vi "Camera_Config.vi"(5 "Crop?":bool, 6 "Camera":T5, 7 "error in":errorcluster, 8 "input cluster":T1={"L16 Linear Actuator"="", "XE 1000 Pump"="", "Camera1"="", "Camera2"="", "Img_Capt"=FALSE, "Actuator"=FALSE, "Pump"=FALSE, "Cam 1"=FALSE, "Cam 2"=FALSE, "Empty_Refill"=FALSE, "Crop"=FALSE, "Light intensity"=100, "Exposure Time"=1000.0, "Sample Name"="Test Sample", "Operator"="MRJ", "Calibration 1"=path "C:/Users/au540322/Desktop/IHS_Project/images/Debris/Debris_0/Debris_0_2019_06_01-23-32-49-686.PNG", "Calibration 2"=path "C:/Users/au540322/Desktop/IHS_Project/images/Debris/Debris_0/Debris_0_2019_06_01-23-32-49-686.PNG", "Framerate"=1, "Timeout Sample"=0, "Collection date"="MRJ", "Sample size threshold"=1, "Empty start"=1, "Command"="MRJ", "Station"="", "Species Name"="", "Other Notes"="", "Aperture"=enum."Item 0", "Image Process Queue Size"=500, "Image Save Queue Size"=500, "Overload threshold"=500, "Max Framerate"=100, "Rectangle 1"={"Left"=0, "Top"=0, "Right"=0, "Bottom"=0, "Rotation"=0.0}, "Rectangle 2"={"Left"=0, "Top"=0, "Right"=0, "Bottom"=0, "Rotation"=0.0}, "Detection Region %"=0.0, "Detect 1"=path "C:/Users/au540322/Desktop/IHS_Project/images/Debris/Debris_0/Debris_0_2019_06_01-23-32-49-686.PNG", "Detect 2"=path "C:/Users/au540322/Desktop/IHS_Project/images/Debris/Debris_0/Debris_0_2019_06_01-23-32-49-686.PNG", "Max large object threshold"=0, "Open(T)/Close(F)"=FALSE, "Img_Capt Begin"=FALSE, "Dispense Speed"=100, "Flush Size"=100, "Location"="Station", "Latitude"="Station", "Longitude"="Station", "Determiner"="Station", "Sex"="Station", "Camera1_Img"=refnum, "Camera2_Img"=refnum, "Img1_Orig_Disp"=refnum, "Img2_Orig_Disp"=refnum, "Img1_Orig_RGB"=refnum, "Img2_Orig_RGB"=refnum, "Blue_Plane_Extract"=refnum, "Subtracted_Plane"=refnum, "Img1_Binary"=refnum, "Img2_Binary"=refnum, "Crop_Mask"=refnum, "Img1_Save"=refnum, "Img2_Save"=refnum, "Img1_Cali_Full"=refnum, "Img2_Cali_Full"=refnum, "Img1_Cali_Detect"=refnum, "Img2_Cali_Detect"=refnum, "Cam 1 queue"=refnum, "Cam 2 queue"=refnum, "Cam 1 - save queue"=refnum, "Cam 2 - save queue"=refnum, "Overlay_Ring"=0, "SystemVersion"=0, "System Serial"=""} {"SystemVersion" items=["Standard", "XL"]; "Overlay_Ring" items=["Session Data", "Extended Setup", "Buffer", "Camera", "Dispenser", "Stats", "Connections"]; "Flush Size" min=1; "Dispense Speed" min=1; "Rectangle 2"."Rotation" format="%.2f"; "Rectangle 2"."Left" scale=0.0..1024.0; "Rectangle 2"."Right" scale=0.0..1024.0; "Rectangle 1"."Rotation" format="%.2f"; "Rectangle 1"."Left" scale=0.0..1024.0; "Rectangle 1"."Right" scale=0.0..1024.0; "Max Framerate" min=1; "Overload threshold" min=1; "Image Save Queue Size" min=1; "Image Process Queue Size" min=1; "Empty start" min=1; "Sample size threshold" min=1; "Framerate" min=1; "Light intensity" scale=0.0..100.0}, 9 "Detect Movement":bool, 10 "Refnum in":T2="cam2") -> (0 "error out":errorcluster, 3 "Refnum out":T2="cam2")   [LabVIEW 2021]
doc: "Configures basler cameras for image acquisition with cropped aspectratio."
uses:
  <vilib>/userDefined/High Color/IMAQdx.ctl
  Camera_ID.ctl
  controls/Data.ctl
  <vilib>/vision/Image Controls.llb/IMAQ Image.ctl
  <resource>/objmgr/imaqdx.rc
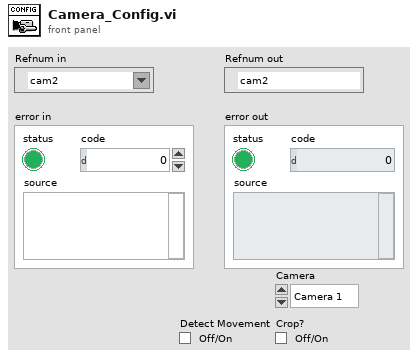
[diagram p1: front panel]
types:
  T1 = typedef "Data.ctl" = cluster{"L16 Linear Actuator":refnum<visa-resource-name>, "XE 1000 Pump":refnum<visa-resource-name>, "Camera1":T2, "Camera2":T2, "Img_Capt":bool, "Actuator":bool, "Pump":bool, "Cam 1":bool, "Cam 2":bool, "Empty_Refill":bool, "Crop":bool, "Light intensity":i32, "Exposure Time":dbl, "Sample Name":string, "Operator":string, "Calibration 1":path, "Calibration 2":path, "Framerate":i32, "Timeout Sample":i32, "Collection date":string, "Sample size threshold":i32, "Empty start":u32, "Command":string, "Station":string, "Species Name":string, "Other Notes":string, "Aperture":enum32{"Item 0", "Item 1", "Item 2", "Item 3"}, "Image Process Queue Size":i32, "Image Save Queue Size":i32, "Overload threshold":i32, "Max Framerate":i32, "Rectangle 1":T3, "Rectangle 2":T3, "Detection Region %":dbl, "Detect 1":path, "Detect 2":path, "Max large object threshold":i32, "Open(T)/Close(F)":bool, "Img_Capt Begin":bool, "Dispense Speed":i32, "Flush Size":i32, "Location":string, "Latitude":string, "Longitude":string, "Determiner":string, "Sex":string, "Camera1_Img":T4, "Camera2_Img":T4, "Img1_Orig_Disp":T4, "Img2_Orig_Disp":T4, "Img1_Orig_RGB":T4, "Img2_Orig_RGB":T4, "Blue_Plane_Extract":T4, "Subtracted_Plane":T4, "Img1_Binary":T4, "Img2_Binary":T4, "Crop_Mask":T4, "Img1_Save":T4, "Img2_Save":T4, "Img1_Cali_Full":T4, "Img2_Cali_Full":T4, "Img1_Cali_Detect":T4, "Img2_Cali_Detect":T4, "Cam 1 queue":refnum<queue>, "Cam 2 queue":refnum<queue>, "Cam 1 - save queue":refnum<queue>, "Cam 2 - save queue":refnum<queue>, "Overlay_Ring":u16, "SystemVersion":u16, "System Serial":string}
  T2 = typedef "IMAQdx.ctl" = refnum<k21>
  T3 = typedef "IMAQ Rectangle" = cluster{"Left":i32, "Top":i32, "Right":i32, "Bottom":i32, "Rotation":dbl}
  T4 = typedef "IMAQ Image.ctl" = refnum<image>
  T5 = typedef "Camera_ID.ctl" = enum16{"Camera 1", "Camera 2"}
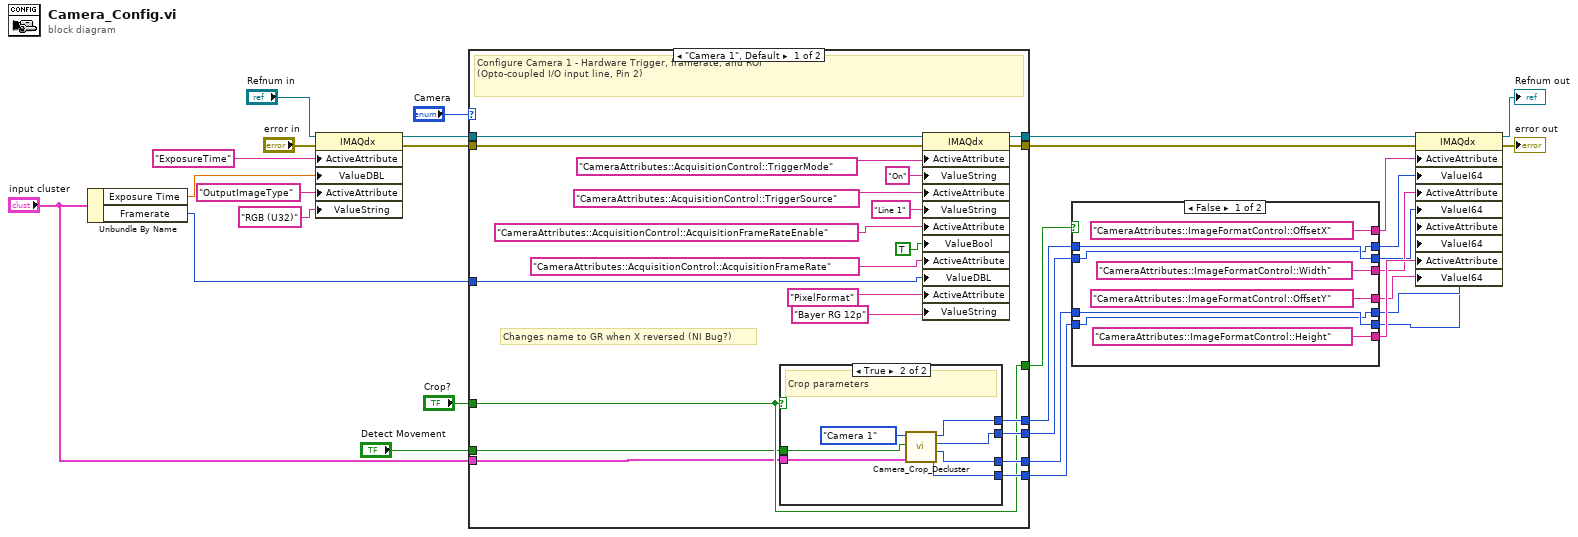
[diagram p0: block diagram]
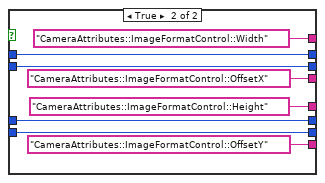
[diagram p2: hidden frame]
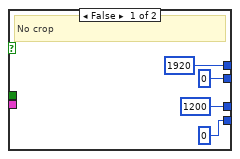
[diagram p3: hidden frame]
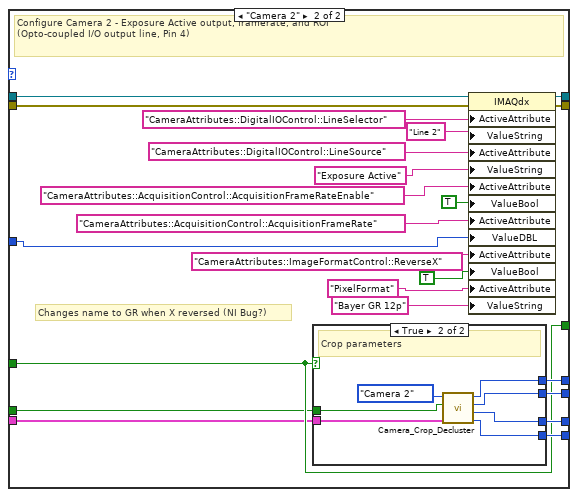
[diagram p4: hidden frame]
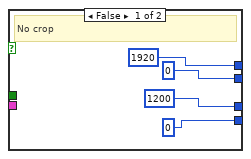
[diagram p5: hidden frame]
diagram:
  n1 = Unbundle By Name("input cluster") -> ("Exposure Time"=w28:dbl, "Framerate"=w27:i32)
  n2 = property class="IMAQdx"(reference="Refnum in", error in="error in", "ActiveAttribute"="ExposureTime", "ValueDBL"=w28, "ActiveAttribute"="OutputImageType", "ValueString"="RGB (U32)") -> (reference out=w21:T2, error out=w3:errorcluster)
  n3 = case shown="\"Camera 1\", Default" "Camera" {
    tunnel: w21 -> [w51 w72]
    tunnel: [w50 w71] -> w19
    tunnel: [w49 w70] -> w26
    tunnel: w27 -> [w41 w69]
    tunnel: [w39 w85] -> w13
    tunnel: [w40 w84] -> w16
    tunnel: [w37 w82] -> w11
    tunnel: [w38 w83] -> w15
    tunnel: "Crop?" -> [w36 w81]
    tunnel: [w36 w81] -> w18
    tunnel: "input cluster" -> [w35 w80]
    tunnel: "Detect Movement" -> [w34 w79]
    tunnel: w3 -> [w33 w65]
    frame "Camera 1", Default {
      # "Changes name to GR when X reversed (NI Bug?)"
      # "Configure Camera 1 - Hardware Trigger, framerate, and ROI \n(Opto-coupled I/O input line, Pin 2)"
      n4 = case shown="True" w36 {
        tunnel: [i64 1920 w61] -> w40
        tunnel: [1200 w59] -> w39
        tunnel: [i64 0 w60] -> w38
        tunnel: [0 w58] -> w37
        tunnel: w35 -> [_ w57]
        tunnel: w34 -> [_ w56]
        frame False {
          # "No crop"
        }
        frame True {
          # "Crop parameters"
          n5 = call "Camera_Crop_Decluster.vi"("input cluster"=w57, "Detect Movement"=w56, "Camera"=Camera_ID."Camera 1") -> ("OffsetY"=w58:i64, "Height"=w59:i64, "OffsetX"=w60:i64, "Width"=w61:i64)  [unwired: 5 in]
        }
      }
      n6 = property class="IMAQdx"(reference=w51, error in=w33, "ActiveAttribute"="CameraAttributes::AcquisitionControl::TriggerMode", "ValueString"="On", "ActiveAttribute"="CameraAttributes::AcquisitionControl::TriggerSource", "ValueString"="Line 1", "ActiveAttribute"="CameraAttributes::AcquisitionControl::AcquisitionFrameRateEnable", "ValueBool"=TRUE, "ActiveAttribute"="CameraAttributes::AcquisitionControl::AcquisitionFrameRate", "ValueDBL"=w41, "ActiveAttribute"="PixelFormat", "ValueString"="Bayer RG 12p") -> (reference out=w50:T2, error out=w49:errorcluster)
    }
    frame "Camera 2" {
      # "Changes name to GR when X reversed (NI Bug?)"
      # "Configure Camera 2 - Exposure Active output, framerate, and ROI\n(Opto-coupled I/O output line, Pin 4)"
      n7 = case shown="True" w81 {
        tunnel: [i64 1200 w92] -> w85
        tunnel: [i64 1920 w94] -> w84
        tunnel: [i64 0 w93] -> w83
        tunnel: [i64 0 w91] -> w82
        tunnel: w80 -> [_ w96]
        tunnel: w79 -> [_ w90]
        frame False {
          # "No crop"
        }
        frame True {
          # "Crop parameters"
          n8 = call "Camera_Crop_Decluster.vi"("input cluster"=w96, "Detect Movement"=w90, "Camera"=Camera_ID."Camera 2") -> ("OffsetY"=w91:i64, "Height"=w92:i64, "OffsetX"=w93:i64, "Width"=w94:i64)  [unwired: 5 in]
        }
      }
      n9 = property class="IMAQdx"(reference=w72, error in=w65, "ActiveAttribute"="CameraAttributes::DigitalIOControl::LineSelector", "ValueString"="Line 2", "ActiveAttribute"="CameraAttributes::DigitalIOControl::LineSource", "ValueString"="Exposure Active", "ActiveAttribute"="CameraAttributes::AcquisitionControl::AcquisitionFrameRateEnable", "ValueBool"=TRUE, "ActiveAttribute"="CameraAttributes::AcquisitionControl::AcquisitionFrameRate", "ValueDBL"=w69, "ActiveAttribute"="CameraAttributes::ImageFormatControl::ReverseX", "ValueBool"=TRUE, "ActiveAttribute"="PixelFormat", "ValueString"="Bayer GR 12p") -> (reference out=w71:T2, error out=w70:errorcluster)
    }
  }
  n10 = case shown="False" w18 {
    tunnel: ["CameraAttributes::ImageFormatControl::Height" ("ActiveAttribute") "CameraAttributes::ImageFormatControl::OffsetY" ("ActiveAttribute")] -> w25
    tunnel: ["CameraAttributes::ImageFormatControl::OffsetY" ("ActiveAttribute") "CameraAttributes::ImageFormatControl::Height" ("ActiveAttribute")] -> w24
    tunnel: ["CameraAttributes::ImageFormatControl::Width" ("ActiveAttribute") "CameraAttributes::ImageFormatControl::OffsetX" ("ActiveAttribute")] -> w23
    tunnel: ["CameraAttributes::ImageFormatControl::OffsetX" ("ActiveAttribute") "CameraAttributes::ImageFormatControl::Width" ("ActiveAttribute")] -> w22
    tunnel: [w99 w108] -> w17
    tunnel: w16 -> [w100 w108]
    tunnel: w15 -> [w99 w107]
    tunnel: [w100 w107] -> w14
    tunnel: w13 -> [w98 w106]
    tunnel: [w97 w106] -> w12
    tunnel: w11 -> [w97 w105]
    tunnel: [w98 w105] -> w10
    frame False {
    }
    frame True {
    }
  }
  n11 = property class="IMAQdx"(reference=w19, error in=w26, "ActiveAttribute"=w22, "ValueI64"=w17, "ActiveAttribute"=w23, "ValueI64"=w14, "ActiveAttribute"=w24, "ValueI64"=w12, "ActiveAttribute"=w25, "ValueI64"=w10) -> (reference out=→"Refnum out":T2, error out=→"error out":errorcluster)
